vi "Get - Paths.vi"(0 "reference in":refnum<class "GSwFormDSP.lvclass">, 5 "error in (no error)":errorcluster) -> (11 "Nb Different Paths":i32, 13 "Path Names":string[](array[string]), 14 "reference out":refnum<class "GSwFormDSP.lvclass">, 19 "error out":errorcluster)   [LabVIEW 2020, in "GSwFormDSP.lvclass"]
uses:
  GSwFormDSP.lvclass
  functions/Attribute List.ctl
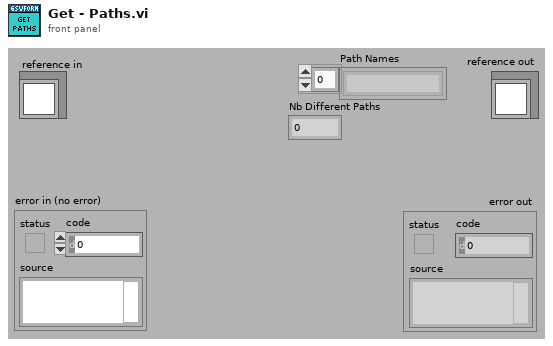
[diagram p1: front panel]
types:
  T1 = typedef "GSwFormDSP.lvclass/Attribute List.ctl" = string
  T2 = typedef "GSwFormDSP.lvclass/ObjectAttributes.ctl" = cluster{"Wform Ref":refnum<data-value>, "Nb Signals":i32, "Spectral Function Parameters":T3, "FFT":waveform(cdb)[], "Nb FFT":i32, "Nb Averages":i32[], "Reference Indexes":i32[], "Response Indexes":i32[], "Coherence":waveform(dbl)[], "TDF Parameters":T5, "DAQ":cluster{"Duration (sec)":dbl, "Buffer Size (Samples)":i32, "Offset (Samples)":i32}, "Filter Impulse Response (TDF)":waveform(dbl), "Sound Playback":T6}
  T3 = typedef "GSwFormDSP.lvclass/Spectral Parameters.ctl" = cluster{"Frequency resolution (Hz)":dbl, "Overlap":dbl, "Window":T4}
  T4 = typedef "NI_AALPro.lvlib/windowTd.ctl" = u32
  T5 = typedef "GSwFormDSP.lvclass/TDF Parameters.ctl" = cluster{"Filter":enum32{"Lowpass", "Highpass", "Bandpass", "Bandstop"}, "Type:":enum16{"Butterworth", "Chebyshev", "Inv Chebyshev", "Elliptic", "Bessel"}, "LP cutoff freq":dbl, "HP cutoff freq":dbl, "Order":i32, "passband ripple (dB)":dbl, "stopband attenuation (dB)":dbl, "Phaseless Filter":bool, "Include Fade IN and OUT":bool}
  T6 = typedef "GSwFormDSP.lvclass/Sound Playback.ctl" = cluster{"Timer start (ms)":u32, "task ID":T7, "Cursor Init Location (s)":dbl, "SC Volume":dbl}
  T7 = typedef "Sound Output Task ID.ctl" = u32
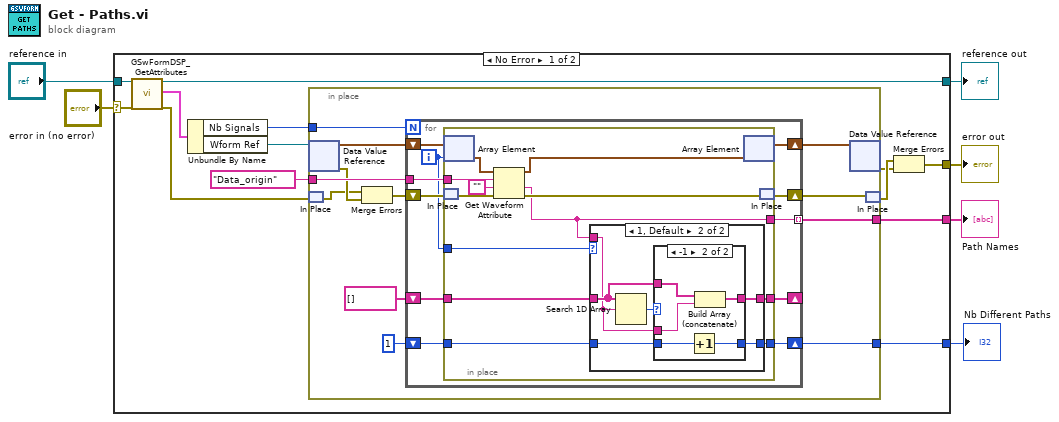
[diagram p0: block diagram]
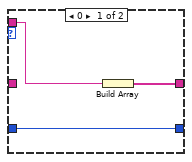
[diagram p2: hidden frame]
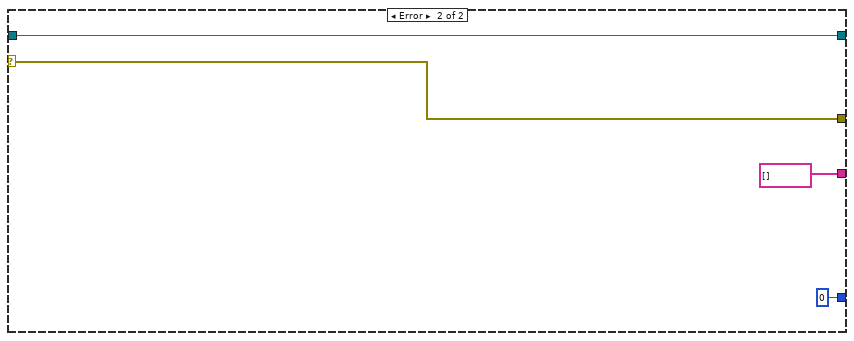
[diagram p4: hidden frame]
diagram:
  n1 = case shown="No Error" "error in (no error)" {
    selector: "error in (no error)" -> [w19 w74]
    tunnel: [w9 w74] -> w5
    tunnel: [w18 w73] -> w3
    tunnel: "reference in" -> [w17 w73]
    tunnel: [w13 string[] []] -> w2
    tunnel: [w7 0] -> w1
    frame No Error {
      n2 = call "GSwFormDSP_GetAttributes.vi"("reference in"=w17, "error in (no error)"=w19) -> ("reference out"=w18:refnum<class "GSwFormDSP.lvclass">, "attributes"=w16:T2, "error out"=w12:errorcluster)  [unwired: 14 in, 1 out]
      n3 = Unbundle By Name(w16) -> ("Nb Signals"=w8:i32, "Wform Ref"=w15:refnum<data-value>)
      n4 = in-place {
        in-place-border: T1 "Data_origin" ("wForm Attributes") -> [w31]
        in-place-border: [w30] -> w13
        in-place-border: w8 -> [w29]
        in-place-border: [w20] -> w7
        n5 = in-place-dvr #1(w15) -> (w28:waveform(dbl)[], w26:errorcluster)
        n6 = in-place-match #2(w12) -> (w24:errorcluster)
        n7 = Merge Errors(w24, w26) -> (w25:errorcluster)
        n8 = for {
          N: w29 -> [_]
          tunnel: [w41] -> w30 mode=indexing
          tunnel: w31 -> [w42]
          shift-right: [w37] -> w23
          shift-left: w25 -> [w38]
          shift-right: [w39] -> w27
          shift-left: w28 -> [w40]
          shift-right: [w33] -> _
          shift-left: string[] [] -> [w32]
          shift-right: [w35] -> w20
          shift-left: 1 -> [w34]
          i -> [w36]
          n9 = in-place {
            in-place-border: w42 -> [w54]
            in-place-border: [w45] -> w41
            in-place-border: w36 -> [w48]
            in-place-border: [w47] -> w35
            in-place-border: w34 -> [w46]
            in-place-border: [w44] -> w33
            in-place-border: w32 -> [w43]
            n10 = in-place-array #3(w40, w36) -> (w52:waveform(dbl))
            n11 = in-place-match #4(w38) -> (w50:errorcluster)
            n12 = Get Waveform Attribute(4:w50, 5:"", 6:w54, 7:w52) -> (0:w49:errorcluster, 1:w45:string, 3:w51:waveform(dbl))  [unwired: 1 out]
            n13 = case shown="1, Default" w48 {
              tunnel: [w57 w60] -> w47
              tunnel: w46 -> [w57 w59]
              tunnel: w45 -> [w56 w58]
              tunnel: [w55 w62] -> w44
              tunnel: w43 -> [_ w61]
              frame 0 {
                n14 = Build Array(w56) -> (w55:string[])
              }
              frame 1, Default {
                n15 = Search 1D Array(1D array=w61, element=w58) -> (index of element=w63:i32)  [unwired: 1 in]
                n16 = case shown="-1" w63 {
                  tunnel: [w65 w66] -> w62
                  tunnel: w61 -> [w65 w70]
                  tunnel: [w64 w68] -> w60
                  tunnel: w59 -> [w64 w69]
                  tunnel: w58 -> [_ w67]
                  frame 0, Default {
                  }
                  frame -1 {
                    n17 = Increment(x=w69) -> (x+1=w68:i32)
                    n18 = Build Array (concatenate)(w70, w67) -> (w66:string[])
                  }
                }
              }
            }
            n19 = in-place-array #3(w51) -> (w39:waveform(dbl)[])  [unwired: 1 out]
            n20 = in-place-match #4(w49) -> (w37:errorcluster)
          }
        }
        n21 = in-place-dvr #1(w27) -> (w10:errorcluster)  [unwired: 1 out]
        n22 = in-place-match #2(w23) -> (w11:errorcluster)
      }
      n23 = Merge Errors(w11, w10) -> (w9:errorcluster)
    }
    frame Error {
    }
  }
  "error out" <- w5
  "reference out" <- w3
  "Path Names" <- w2
  "Nb Different Paths" <- w1
